vi "dsymm - Symmetric Matrix-Matrix Product (DBL).vi"(4 "beta":dbl=1.0, 5 "side":T2=1 items=["Left"=1, "Right"=0], 6 "alpha":dbl=1.0, 8 "matrix A type":T1=3 items=["Lower Triangular"=2, "Upper Triangular"=3], 9 "C":T3, 10 "B":T3, 11 "A":T3) -> (0 "error":i32, 3 "dsymm":T3)   [LabVIEW 2020, in "NI_AALBLAS.lvlib"]
doc: "Calculates the product of a symmetric matrix and another matrix."
uses:
  <vilib>/Analysis/NI_AALBLAS.lvlib
  <vilib>/Analysis/Matrix/Datatypes/RealMatrix.ctl
  <vilib>/Analysis/BLAS.llb/LV_Side.ctl
  <vilib>/Analysis/BLAS.llb/LV_UpLo.ctl
  <vilib>/Analysis/BLAS.llb/Fucntion.ctl
  <vilib>/Analysis/BLAS.llb/Order.ctl
  <vilib>/Analysis/BLAS.llb/BLAS3 Utility(DBL).vi
  <vilib>/Analysis/Matrix/NI_Matrix.lvlib
panel:
  # "dsymm=alpha*A*B+beta*C / dsymm=alpha*B*A+beta*C"
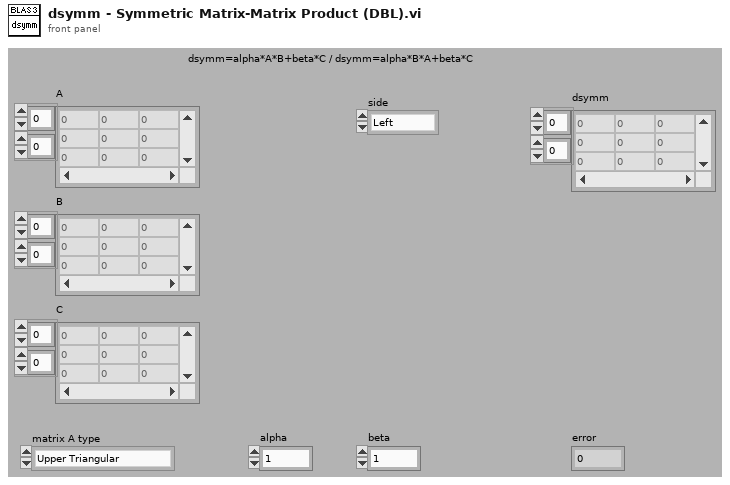
[diagram p1: front panel]
types:
  T1 = typedef "NI_AALBLAS.lvlib/LV_UpLo.ctl" = i32
  T2 = typedef "NI_AALBLAS.lvlib/LV_Side.ctl" = i32
  T3 = typedef "NI_Matrix.lvlib/RealMatrix.ctl" = dbl[][]
  T4 = typedef "NI_AALBLAS.lvlib/Order.ctl" = i32
  T5 = typedef "NI_AALBLAS.lvlib/Fucntion.ctl" = u16
  T6 = typedef "NI_AALBLAS.lvlib/UpLo.ctl" = i32
  T7 = typedef "NI_AALBLAS.lvlib/Side.ctl" = i32
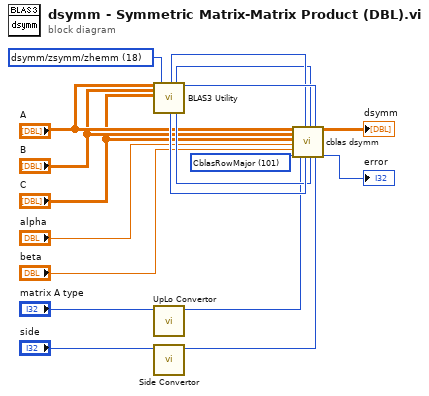
[diagram p0: block diagram]
diagram:
  w1 = T4 101 items=["CblasRowMajor"=101, "CblasColMajor"=102] ("order")
  w5 = T5 18 items=["ddot/zdotu/zdotc", "daxpy/zaxpy", "dnrm2/dznrm2", "dasum/dzasum", "dcopy/zcopy", "dswap/zswap", "drotm", "drot/zdrot", "idamax/izamax", "idamin/izamin", "dgemv/zgemv", "dsymv/zhemv", "dtrmv/ztrmv", "dsyr/zher", "dsyr2/zher2", "dger/zgeru/zgerc", "dtrsv/ztrsv", "dgemm/zgemm", "dsymm/zsymm/zhemm", "dtrmm/ztrmm", "dsyrk/zsyrk/zherk", "dsyr2k/zsyr2k/zher2k", "dtrsm/ztrsm"] ("function")
  n1 = call-poly <vilib>:"BLAS3 Utility.vi"("A"="A", "B/X"="B", "C"="C", "function"=w5) -> ("lda"=w3:i32, "m"=w18:i32, "ldb/ldx"=w2:i32, "n"=w17:i32, "ldc"=w4:i32)  [unwired: 2 in, 9 out]
  n2 = call <vilib>:"UpLo Convertor.vi"("triangle matrix type"="matrix A type") -> ("uplo"=w13:T6)  [unwired: 10 out]
  n3 = call <vilib>:"Side Convertor.vi"("LV side"="side") -> ("side"=w11:T7)  [unwired: 10 out]
  n4 = call <vilib>:"cblas dsymm.vi"("A"="A", "B"="B", "C"="C", "alpha"="alpha", "beta"="beta", "order"=w1, "uplo"=w13, "lda"=w3, "m"=w18, "ldb"=w2, "n"=w17, "ldc"=w4, "side"=w11) -> ("dsymm"=→"dsymm":T3, "error"=→"error":i32)  [unwired: 5 out]
